vi "Save Bundle Definitions.vi"(8 "error in (no error)":errorcluster, 11 "Bundle Builder in":refnum<class "Bundle Builder.lvclass">) -> (0 "error out":errorcluster, 3 "Bundle Builder out":refnum<class "Bundle Builder.lvclass">)   [LabVIEW 2020, in "Bundle Builder.lvclass"]
uses:
  Bundle Builder.lvclass
  Bundle Builder.lvclass/Bundle Builder.ctl
  C:/Users/chihong/Documents/Repos/StsCustomBundleBuilder/Code/StsCustomBundleBuilder/StsCustomBundleBuilderLib/StsCustomBundleBuilderLib.dll
  StsCustomBundleBuilderLib/StsCustomBundleBuilderLib.dll
  <vilib>/Utility/error.llb/Error Cluster From Error Code.vi
  <vilib>/ErrorRing/Error Ring.xnode
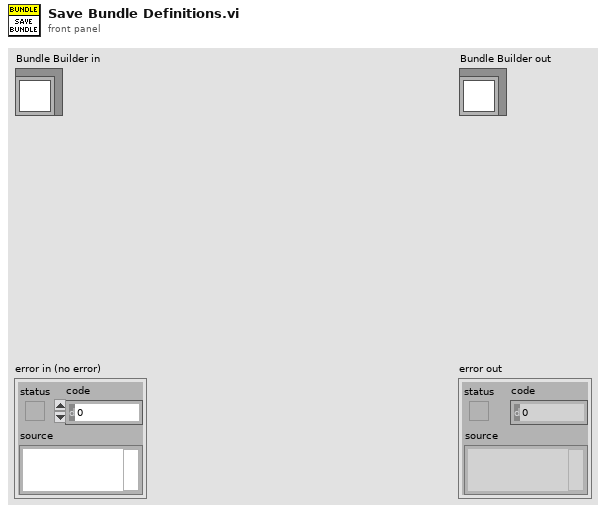
[diagram p1: front panel]
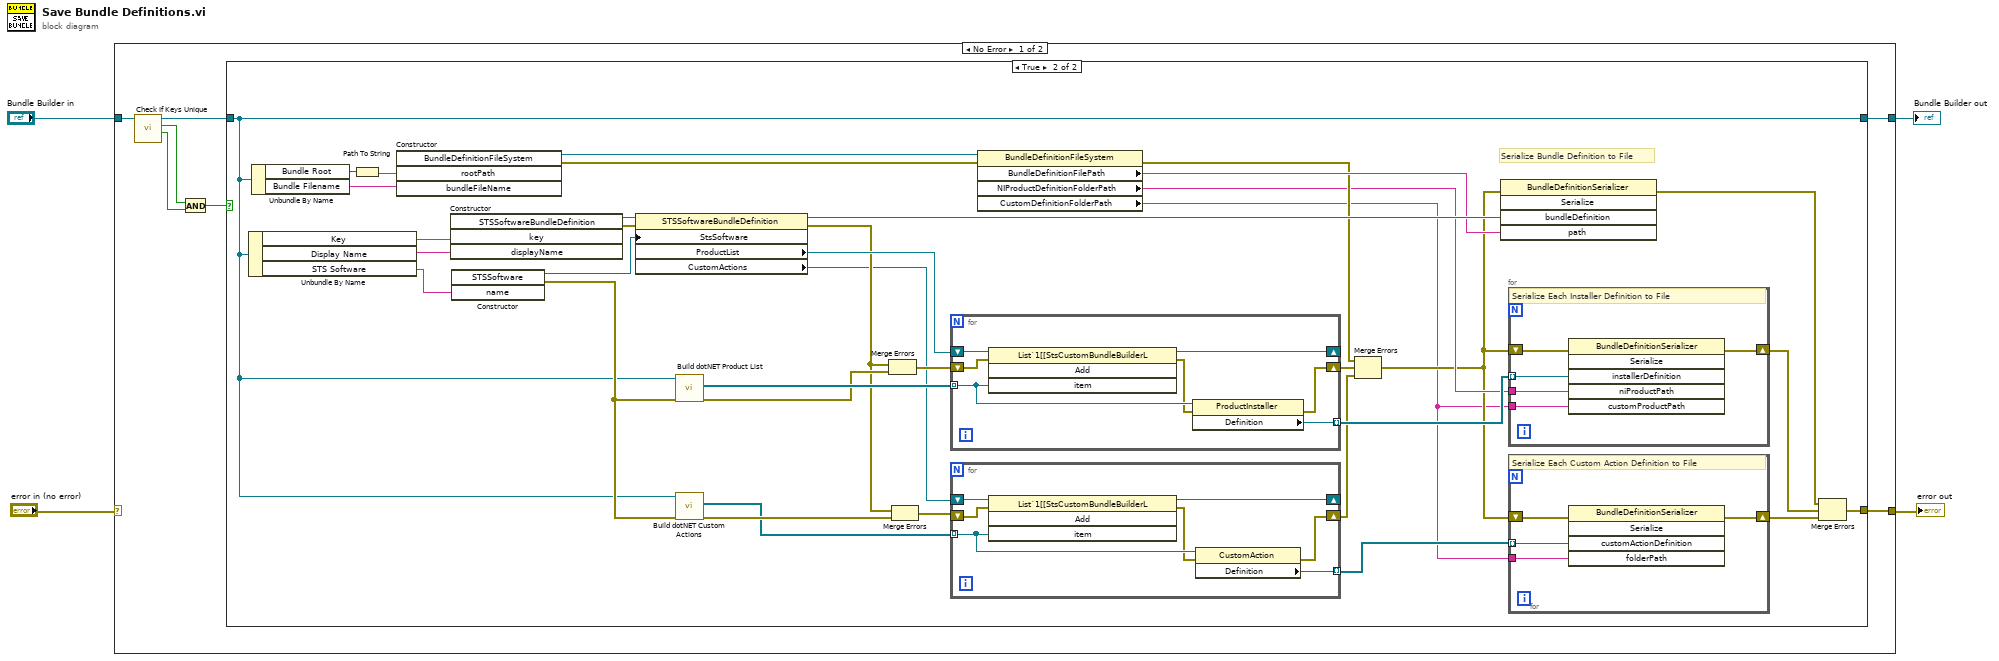
[diagram p0: block diagram]
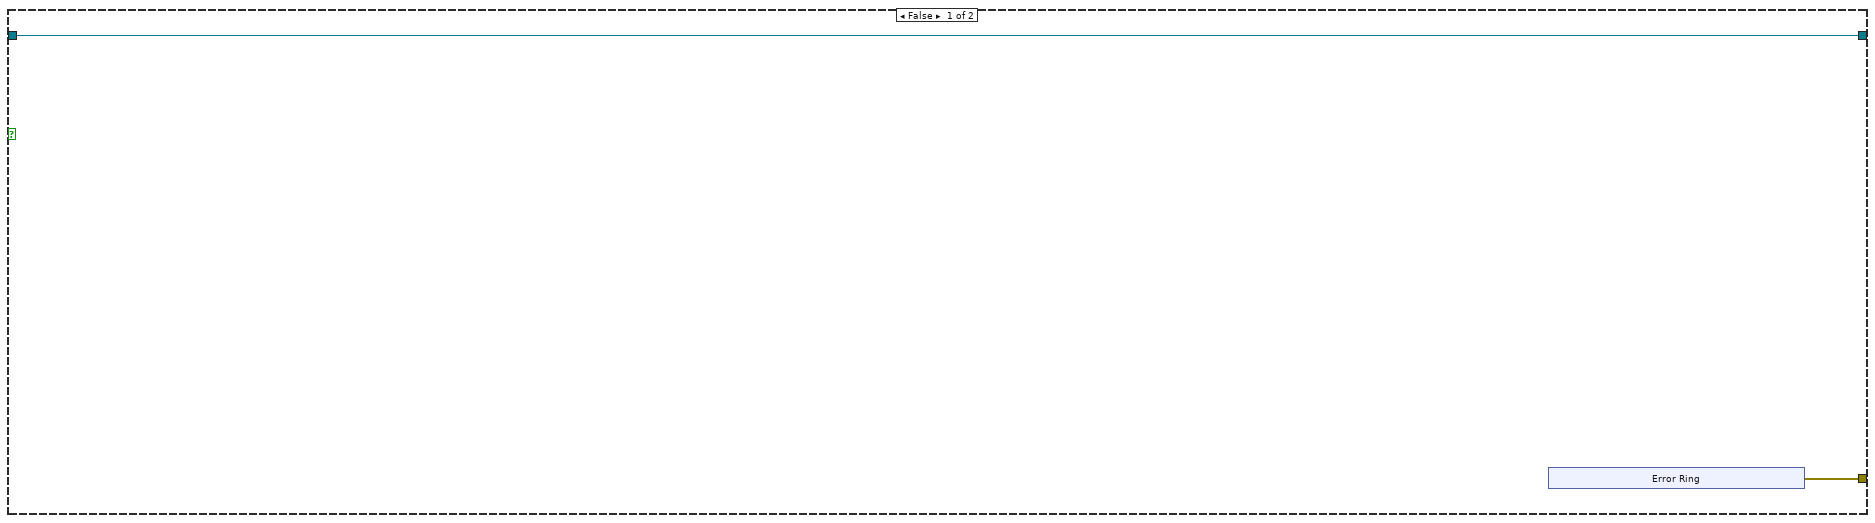
[diagram p2: hidden frame]
diagram:
  n1 = case shown="No Error" "error in (no error)" {
    selector: "error in (no error)" -> [_ w79]
    tunnel: [w5 w79] -> w3
    tunnel: [w6 w78] -> w1
    tunnel: "Bundle Builder in" -> [w11 w78]
    frame No Error {
      n2 = call "Check If Keys Unique.vi"("Bundle Builder in"=w11) -> ("Custom Action Key Unique?"=w9:bool, "Product Key Unique?"=w10:bool, "Bundle Builder out"=w7:refnum<class "Bundle Builder.lvclass">)  [unwired: 7 in, 1 out]
      n3 = And(x=w10, y=w9) -> (x .and. y?=w8:bool)
      n4 = case shown="True" w8 {
        tunnel: w7 -> [w13 w19]
        tunnel: [w13 w19] -> w6
        tunnel: [w12 w20] -> w5
        frame False {
          n5 = xnode "Error Ring"() -> ("error out"=w12:errorcluster)
        }
        frame True {
          # "Serialize Bundle Definition to File"
          n6 = Unbundle By Name(w19) -> ("Key"=w50:string, "Display Name"=w49:string, "STS Software"=w48:string)
          n7 = Unbundle By Name(w19) -> ("Bundle Root"=w54:path, "Bundle Filename"=w52:string)
          n8 = Path To String(path=w54) -> (string=w53:string)
          n9 = constructor class="BundleDefinitionFileSystem"("rootPath"=w53, "bundleFileName"=w52) -> (reference out=w36:refnum<k24>, error out=w32:errorcluster)  [unwired: 3 in, 3 out]
          n10 = constructor class="STSSoftwareBundleDefinition"("key"=w50, "displayName"=w49) -> (reference out=w51:refnum<k24>, error out=w44:errorcluster)  [unwired: 3 in, 3 out]
          n11 = constructor class="STSSoftware"("name"=w48) -> (reference out=w47:refnum<k24>, error out=w42:errorcluster)  [unwired: 3 in, 2 out]
          n12 = property class="STSSoftwareBundleDefinition"(reference=w51, error in=w44, "StsSoftware"=w47) -> (reference out=w37:refnum<k24>, error out=w39:errorcluster, "ProductList"=w46:refnum<k24>, "CustomActions"=w29:refnum<k24>)
          n13 = call "Build dotNET Product List.vi"("error in (no error)"=w42, "Bundle Builder in"=w19) -> ("error out"=w43:errorcluster, "Product List"=w45:refnum<k24>[])  [unwired: 7 in, 1 out]
          n14 = call "Build dotNET Custom Actions.vi"("error in (no error)"=w42, "Bundle Builder in"=w19) -> ("error out"=w41:errorcluster, "Custom Actions"=w28:refnum<k24>[])  [unwired: 7 in, 1 out]
          n15 = Merge Errors(w39, w43) -> (w40:errorcluster)
          n16 = Merge Errors(w39, w41) -> (w30:errorcluster)
          n17 = for {
            tunnel: w45 -> [w74] mode=indexing
            shift-right: [w71] -> w38
            shift-left: w40 -> [w76]
            shift-right: [w75] -> _
            shift-left: w46 -> [w77]
            tunnel: [w73] -> w33 mode=indexing
            n18 = invoke class="List`1[[StsCustomBundleBuilderL" method="Add"(reference=w77, error in=w76, "item"=w74) -> (reference out=w75:refnum<k24>, error out=w72:errorcluster)  [unwired: 1 in, 2 out]
            n19 = property class="ProductInstaller"(reference=w74, error in=w72) -> (error out=w71:errorcluster, "Definition"=w73:refnum<k24>)  [unwired: 1 out]
          }
          n20 = for {
            tunnel: w28 -> [w62] mode=indexing
            shift-right: [w59] -> w27
            shift-left: w30 -> [w64]
            shift-right: [w63] -> _
            shift-left: w29 -> [w65]
            tunnel: [w61] -> w25 mode=indexing
            n21 = invoke class="List`1[[StsCustomBundleBuilderL" method="Add"(reference=w65, error in=w64, "item"=w62) -> (reference out=w63:refnum<k24>, error out=w60:errorcluster)  [unwired: 1 in, 2 out]
            n22 = property class="CustomAction"(reference=w62, error in=w60) -> (error out=w59:errorcluster, "Definition"=w61:refnum<k24>)  [unwired: 1 out]
          }
          n23 = property class="BundleDefinitionFileSystem"(reference=w36, error in=w32) -> (error out=w34:errorcluster, "BundleDefinitionFilePath"=w35:string, "NIProductDefinitionFolderPath"=w31:string, "CustomDefinitionFolderPath"=w24:string)  [unwired: 1 out]
          n24 = Merge Errors(w34, w38, w27) -> (w26:errorcluster)
          n25 = invoke class="BundleDefinitionSerializer" method="Serialize"(error in=w26, "bundleDefinition"=w37, "path"=w35) -> (error out=w23:errorcluster)  [unwired: 2 in, 4 out]
          n26 = for {
            tunnel: w33 -> [w70] mode=indexing
            tunnel: w31 -> [w68]
            tunnel: w24 -> [w67]
            shift-right: [w66] -> w22
            shift-left: w26 -> [w69]
            # "Serialize Each Installer Definition to File"
            n27 = invoke class="BundleDefinitionSerializer" method="Serialize"(error in=w69, "installerDefinition"=w70, "niProductPath"=w68, "customProductPath"=w67) -> (error out=w66:errorcluster)  [unwired: 2 in, 5 out]
          }
          n28 = for {
            tunnel: w25 -> [w58] mode=indexing
            tunnel: w24 -> [w56]
            shift-right: [w55] -> w21
            shift-left: w26 -> [w57]
            # "Serialize Each Custom Action Definition to File"
            n29 = invoke class="BundleDefinitionSerializer" method="Serialize"(error in=w57, "customActionDefinition"=w58, "folderPath"=w56) -> (error out=w55:errorcluster)  [unwired: 2 in, 4 out]
          }
          n30 = Merge Errors(w23, w22, w21) -> (w20:errorcluster)
        }
      }
    }
    frame Error {
    }
  }
  "error out" <- w3
  "Bundle Builder out" <- w1
